vi "WriteToMasterBatch.vi"(9 "Scan name":string, 10 "Raw_Data Folder":path) -> ()   [LabVIEW 2013]
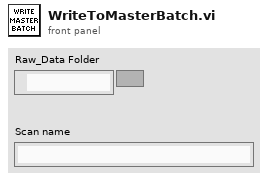
[diagram p1: front panel]
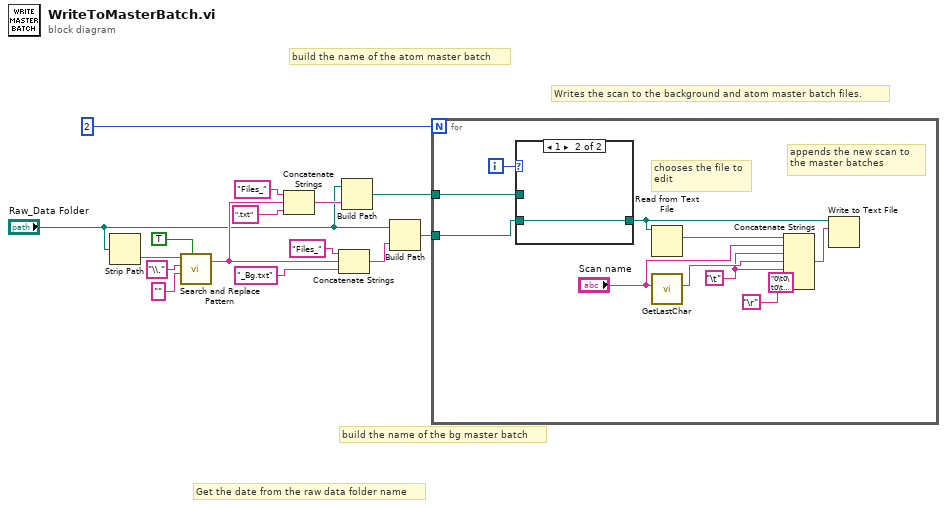
[diagram p0: block diagram]
diagram:
  # "build the name of the bg master batch"
  # "build the name of the atom master batch"
  # "Get the date from the raw data folder name"
  # "Writes the scan to the background and atom master batch files."
  n1 = Strip Path(path="Raw_Data Folder") -> (name=w15:string)  [unwired: 1 out]
  n2 = call <vilib>:"Search and Replace Pattern.vi"("string"=w15, "regular expression (\"\")"="\\." ("regular expression (\"\")"), "replace string (\"\")"="" ("replace string (\"\")"), "replace all? (F)"=TRUE) -> ("result string"=w9:string)  [unwired: 1 in, 1 out]
  n3 = Concatenate Strings("Files_" ("string"), w9, ".txt" ("string")) -> (w6:string)
  n4 = Concatenate Strings("Files_" ("string"), w9, "_Bg.txt" ("string")) -> (w4:string)
  n5 = Build Path(base path="Raw_Data Folder", name or relative path=w6) -> (appended path=w2:path)
  n6 = Build Path(base path="Raw_Data Folder", name or relative path=w4) -> (appended path=w1:path)
  n7 = for {
    N: 2 -> [_]
    tunnel: w2 -> [w25]
    tunnel: w1 -> [w24]
    i -> [w26]
    w18 = "\t"
    # "appends the new scan to \nthe master batches"
    # "chooses the file to\nedit"
    n8 = case shown="1" w26 {
      tunnel: [w27 w28] -> w21
      tunnel: w25 -> [w27 _]
      tunnel: w24 -> [_ w28]
      frame 0, Default {
      }
      frame 1 {
      }
    }
    n9 = Read from Text File(file (use dialog)=w21) -> (text=w23:string)  [unwired: 3 in, 3 out]
    n10 = call "GetLastChar.vi"("String"="Scan name") -> ("String 2"=w19:string)  [unwired: 10 in]
    n11 = Concatenate Strings(w23, "Scan name", w18, w19, w18, "0\t0\t0\t0 \t 27 \t 275 \t 265 \t 500   725" ("string"), "\r") -> (w22:string)
    n12 = Write to Text File(file (use dialog)=w21, text=w22) -> ()  [unwired: 2 in, 3 out]
  }
